vi "CDMA_RxCRC.vi"(8 "error in (no error)":errorcluster caption="错误输入（无错误）", 9 "rx_crc_num":dbl, 10 "ch_decode_data":dbl[](array[numeric]), 11 "Path In":path) -> (0 "error out":errorcluster caption="错误输出", 2 "CRC_flag":dbl, 3 "Path Out":path)   [LabVIEW 2015]
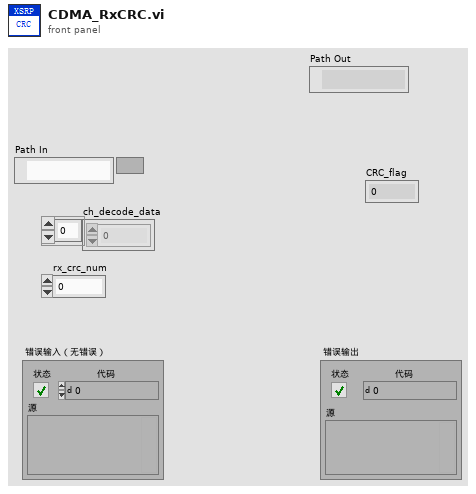
[diagram p1: front panel]
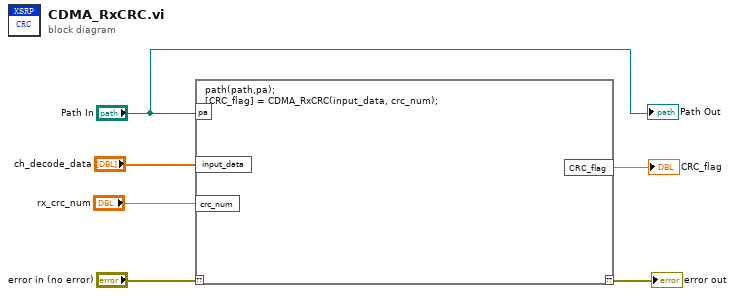
[diagram p0: block diagram]
diagram:
  n1 = script code="path(path,pa);\n[CRC_flag] = CDMA_RxCRC(input_data, crc_num);"("??"="error in (no error)", "pa"="Path In", "input_data"="ch_decode_data", "crc_num"="rx_crc_num") -> ("??"=→"error out":errorcluster, "CRC_flag"=→"CRC_flag":dbl)
  "Path Out" <- "Path In"
